vi "final.vi"() -> ()   [LabVIEW 2022 SP3]
uses:
  <vilib>/DAQmx/write.llb/DAQmx Write (Digital Bool 1Line 1Point).vi
  <vilib>/DAQmx/create/channels.llb/DAQmx Create Channel (DO-Digital Output).vi
  <vilib>/DAQmx/miscellaneous.llb/DAQmx Fill In Error Info.vi
  <vilib>/Instr/_visa.llb/VISA Configure Serial Port (Instr).vi
panel:
  out "read buffer":string
  out "array":dbl[](array[numeric])
  in  "stop":bool
  in  "VISA resource name 2":refnum<visa-resource-name>
  out "Numeric":i32
  out "red":bool
  out "blue":bool
  out "green":bool
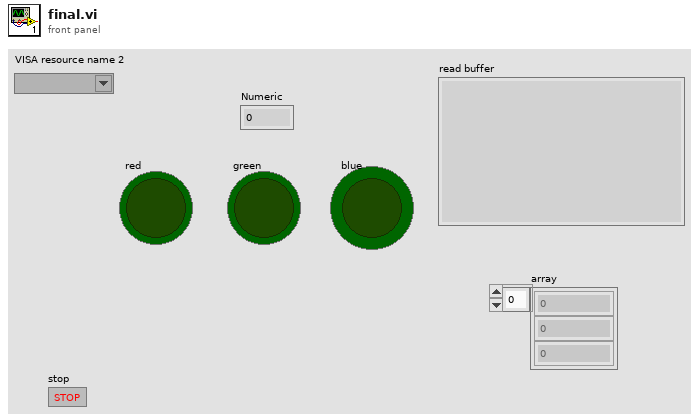
[diagram p1: front panel]
types:
  T1 = cluster{"array type (2D Dbl)[0]":dbl, "array type (2D Dbl)[1]":dbl, "array type (2D Dbl)[2]":dbl}
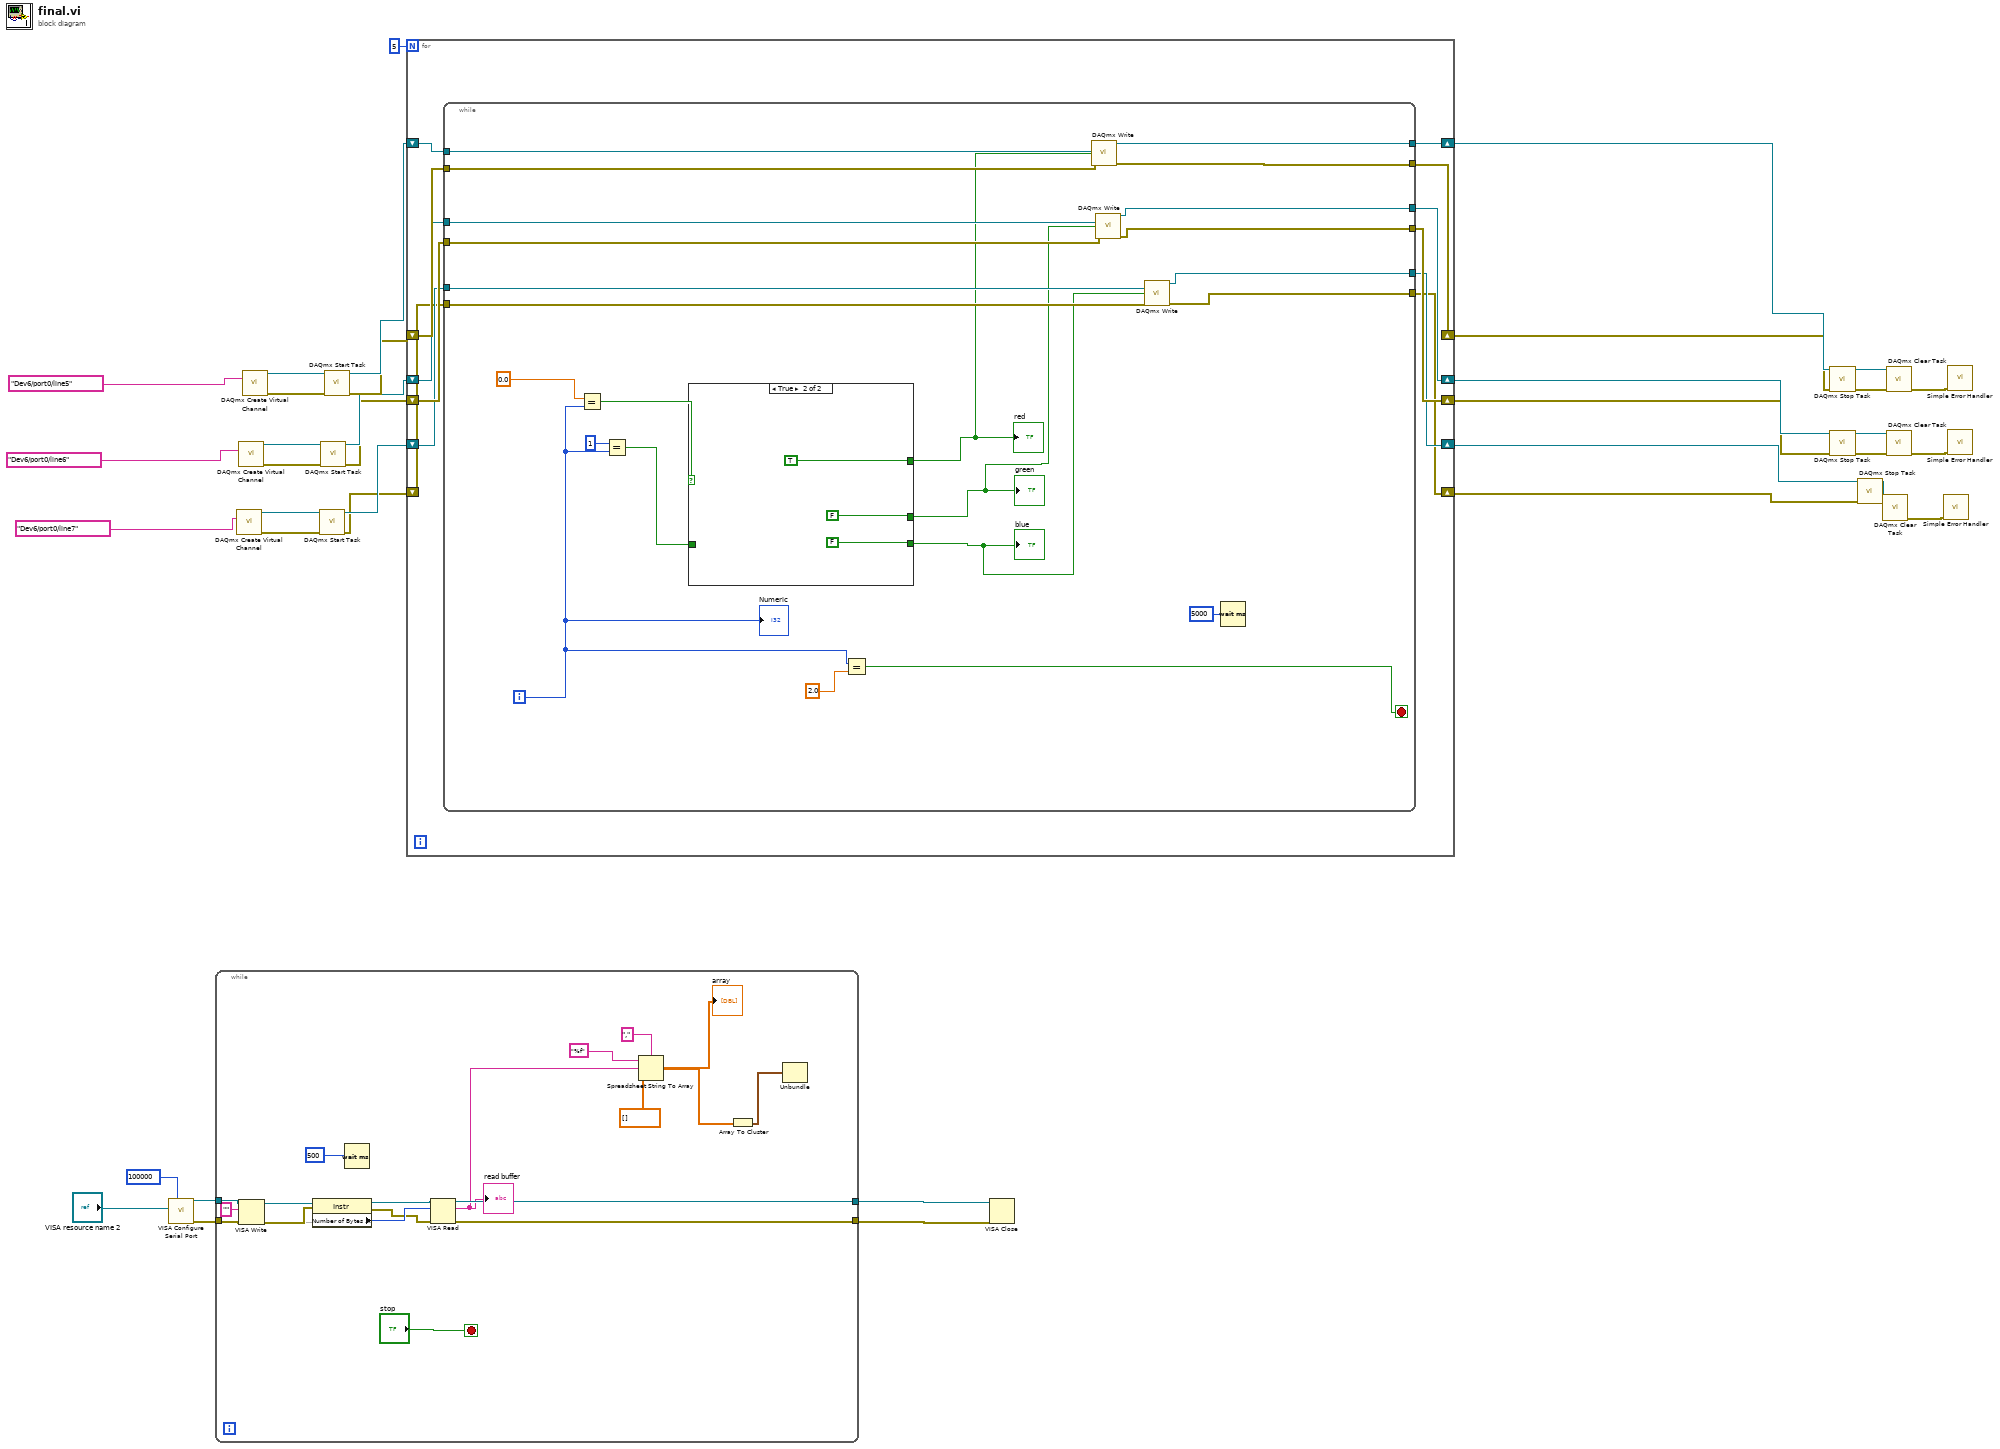
[diagram p0: block diagram]
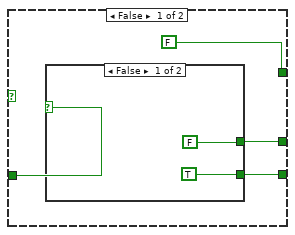
[diagram p2: hidden frame]
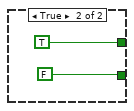
[diagram p3: hidden frame]
diagram:
  n1 = call-poly "VISA Configure Serial Port"("VISA resource name"="VISA resource name 2", "timeout (10sec)"=u32 100000) -> ("VISA resource name out"=w4:refnum<visa-resource-name>, "error out"=w3:errorcluster)  [unwired: 12 in]
  n2 = while {
    tunnel: w4 -> [w55]
    tunnel: w3 -> [w54]
    tunnel: [w48] -> w2
    tunnel: [w47] -> w1
    stop <- "stop" stop-if-true
    n3 = VISA Write(VISA resource name=w55, write buffer="", error in (no error)=w54) -> (VISA resource name out=w53:refnum<visa-resource-name>, error out=w52:errorcluster)  [unwired: 1 out]
    n4 = property class="Instr"(reference=w53, error in=w52) -> (reference out=w50:refnum<visa-resource-name>, error out=w49:errorcluster, "Serial Settings:Number of Bytes at Serial Port"=w51:u32)
    n5 = Wait (ms)(milliseconds to wait=u32 500 ("millisecond timer value")) -> ()  [unwired: 1 out]
    n6 = VISA Read(VISA resource name=w50, byte count=w51, error in (no error)=w49) -> (VISA resource name out=w48:refnum<visa-resource-name>, read buffer=w41:string, error out=w47:errorcluster)  [unwired: 1 out]
    "read buffer" <- w41
    n7 = Spreadsheet String To Array(delimiter (Tab)=",", format string="%f", spreadsheet string=w41, array type (2D Dbl)=dbl[] []) -> (array=w39:dbl[])
    "array" <- w39
    n8 = Array To Cluster(array=w39) -> (cluster=w38:T1)
    n9 = Unbundle(w38) -> ()  [unwired: 3 out]
  }
  n10 = call-poly <vilib>:"DAQmx Create Virtual Channel.vi"("lines"=tag "Dev6/port0/line7" ("Blue Channel")) -> ("task out"=w26:refnum<k21>, "error out"=w27:errorcluster)  [unwired: 13 in]
  n11 = call-poly <vilib>:"DAQmx Create Virtual Channel.vi"("lines"=tag "Dev6/port0/line6" ("Green Channel")) -> ("task out"=w31:refnum<k21>, "error out"=w32:errorcluster)  [unwired: 13 in]
  n12 = call-poly <vilib>:"DAQmx Create Virtual Channel.vi"("lines"=tag "Dev6/port0/line5" ("Red Channel")) -> ("task out"=w36:refnum<k21>, "error out"=w37:errorcluster)  [unwired: 13 in]
  n13 = call <vilib>:"DAQmx Start Task.vi"("task/channels in"=w26, "error in"=w27) -> ("task out"=w15:refnum<k21>, "error out"=w14:errorcluster)  [unwired: 12 in]
  n14 = call <vilib>:"DAQmx Start Task.vi"("task/channels in"=w31, "error in"=w32) -> ("task out"=w17:refnum<k21>, "error out"=w16:errorcluster)  [unwired: 12 in]
  n15 = call <vilib>:"DAQmx Start Task.vi"("task/channels in"=w36, "error in"=w37) -> ("task out"=w19:refnum<k21>, "error out"=w18:errorcluster)  [unwired: 12 in]
  n16 = for {
    N: 5 -> [_]
    shift-right: [w61] -> w13
    shift-left: w19 -> [w67]
    shift-right: [w60] -> w12
    shift-left: w18 -> [w66]
    shift-right: [w59] -> w11
    shift-left: w17 -> [w65]
    shift-right: [w58] -> w10
    shift-left: w16 -> [w64]
    shift-right: [w57] -> w9
    shift-left: w15 -> [w63]
    shift-right: [w56] -> w8
    shift-left: w14 -> [w62]
    n17 = while {
      tunnel: w67 -> [w82]
      tunnel: w66 -> [w81]
      tunnel: [w80] -> w61
      tunnel: [w79] -> w60
      tunnel: w65 -> [w78]
      tunnel: w64 -> [w77]
      tunnel: [w76] -> w59
      tunnel: [w75] -> w58
      tunnel: w63 -> [w74]
      tunnel: w62 -> [w73]
      tunnel: [w72] -> w57
      tunnel: [w71] -> w56
      i -> [w84]
      stop <- w89 stop-if-true
      n18 = Equal?(x=0.0, y=w84) -> (x = y?=w86:bool)
      n19 = Equal?(x=1, y=w84) -> (x = y?=w85:bool)
      n20 = case shown="True" w86 {
        tunnel: [FALSE TRUE] -> w70
        tunnel: w85 -> [w94 _]
        tunnel: [w92 FALSE] -> w69
        tunnel: [w91 FALSE] -> w68
        frame False {
          n21 = case shown="False" w94 {
            tunnel: [FALSE TRUE] -> w92
            tunnel: [TRUE FALSE] -> w91
            frame False {
            }
            frame True {
            }
          }
        }
        frame True {
        }
      }
      "red" <- w70
      "blue" <- w68
      "green" <- w69
      n22 = Equal?(x=w84, y=2.0) -> (x = y?=w89:bool)
      n23 = call-poly <vilib>:"DAQmx Write.vi"("task/channels in"=w82, "data"=w70, "error in"=w81) -> ("task out"=w80:refnum<k21>, "error out"=w79:errorcluster)  [unwired: 10 in, 1 out]
      n24 = call-poly <vilib>:"DAQmx Write.vi"("task/channels in"=w78, "data"=w69, "error in"=w77) -> ("task out"=w76:refnum<k21>, "error out"=w75:errorcluster)  [unwired: 10 in, 1 out]
      n25 = call-poly <vilib>:"DAQmx Write.vi"("task/channels in"=w74, "data"=w68, "error in"=w73) -> ("task out"=w72:refnum<k21>, "error out"=w71:errorcluster)  [unwired: 10 in, 1 out]
      n26 = Wait (ms)(milliseconds to wait=u32 5000) -> ()  [unwired: 1 out]
      "Numeric" <- w84
    }
  }
  n27 = VISA Close(VISA resource name=w2, error in (no error)=w1) -> ()  [unwired: 1 out]
  n28 = call <vilib>:"DAQmx Stop Task.vi"("task/channels in"=w13, "error in"=w12) -> ("task out"=w35:refnum<k21>, "error out"=w34:errorcluster)  [unwired: 12 in]
  n29 = call <vilib>:"DAQmx Stop Task.vi"("task/channels in"=w11, "error in"=w10) -> ("task out"=w30:refnum<k21>, "error out"=w29:errorcluster)  [unwired: 12 in]
  n30 = call <vilib>:"DAQmx Stop Task.vi"("task/channels in"=w9, "error in"=w8) -> ("task out"=w25:refnum<k21>, "error out"=w24:errorcluster)  [unwired: 12 in]
  n31 = call <vilib>:"DAQmx Clear Task.vi"("task in"=w25, "error in"=w24) -> ("error out"=w23:errorcluster)  [unwired: 13 in]
  n32 = call <vilib>:"DAQmx Clear Task.vi"("task in"=w35, "error in"=w34) -> ("error out"=w33:errorcluster)  [unwired: 13 in]
  n33 = call <vilib>:"DAQmx Clear Task.vi"("task in"=w30, "error in"=w29) -> ("error out"=w28:errorcluster)  [unwired: 13 in]
  n34 = call <vilib>:"Simple Error Handler.vi"("error in (no error)"=w23) -> ()  [unwired: 4 in, 5 out]
  n35 = call <vilib>:"Simple Error Handler.vi"("error in (no error)"=w33) -> ()  [unwired: 4 in, 5 out]
  n36 = call <vilib>:"Simple Error Handler.vi"("error in (no error)"=w28) -> ()  [unwired: 4 in, 5 out]
